vi "Load FLAC.vi"(8 "error in (no error)":errorcluster, 11 "Path":path) -> (0 "error out":errorcluster, 1 "data":waveform(i16)[](array[waveform]), 2 "Sample Rate (Hz)":u32, 3 "Channels":u32, 5 "Length (Samples)":u64)   [LabVIEW 2019, in "LabVIEW Audio Codecs.lvlib"]
doc: "Loads a FLAC file from disk.\n\n<b>Priority:</b> Background priority (lowest)"
uses:
  LabVIEW Audio Codecs.lvlib
  labview_audio_codecs_x86.dll
  labview_audio_codecs_x64.dll
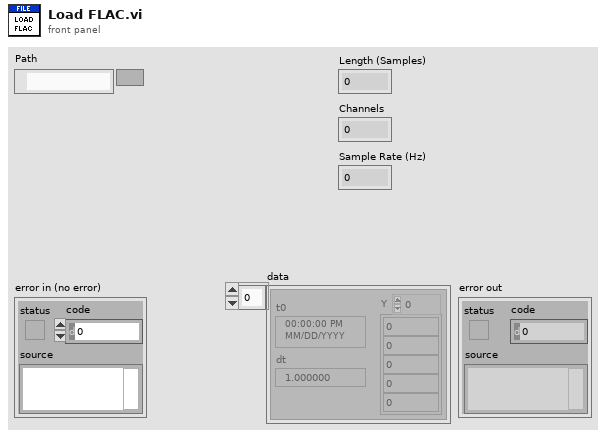
[diagram p1: front panel]
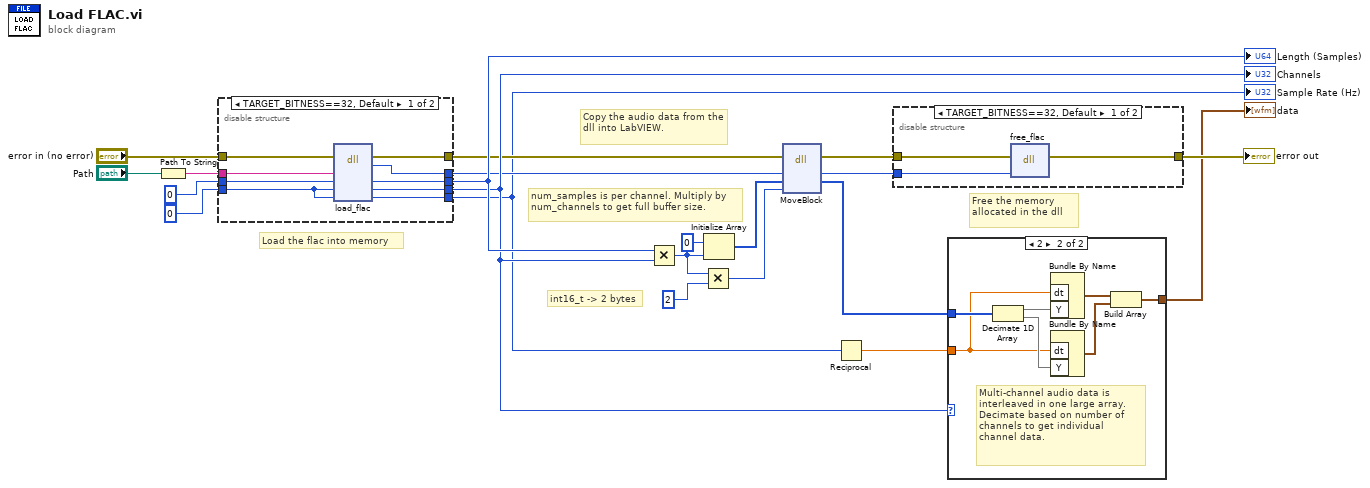
[diagram p0: block diagram]
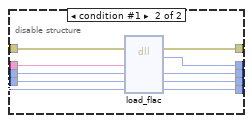
[diagram p2: hidden frame]
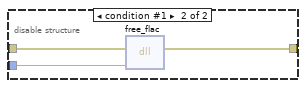
[diagram p3: hidden frame]
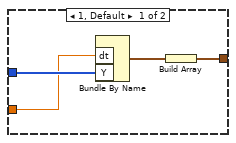
[diagram p4: hidden frame]
diagram:
  # "num_samples is per channel. Multiply by num_channels to get full buffer size."
  # "Free the memory allocated in the dll"
  # "Copy the audio data from the dll into LabVIEW."
  # "Load the flac into memory"
  # "int16_t -> 2 bytes"
  n1 = Path To String(path="Path") -> (string=w15:string)
  n2 = disable-structure shown="TARGET_BITNESS==32, Default" {
    disable-tunnel: "error in (no error)" -> [w30 w39]
    disable-tunnel: [w29 w38] -> w18
    disable-tunnel: [w28 w37] -> w17
    disable-tunnel: [w27 w36] -> w2
    disable-tunnel: w15 -> [w26 w35]
    disable-tunnel: u32 0 ("num_samples") -> [w25 w34]
    disable-tunnel: [w24 w33] -> w12
    disable-tunnel: [w23 w32] -> w10
    disable-tunnel: u64 0 ("num_samples") -> [w22 w31]
    frame condition #0 (active) {
      n3 = dll-call lib="C:/github/dataflowg/labview-simcity-2000-toolkit/src/Sound/LabVIEW Audio Codecs/labview_audio_codecs_x86.*" fn="load_flac"(error in=w30, "file_name"=w26, "num_samples"=w22, "channels"=w25, "sample_rate"=w25) -> (error out=w23:errorcluster, "return type"=w24:i64, "num_samples"=w29:u64, "channels"=w28:u32, "sample_rate"=w27:u32)  [unwired: 3 in, 1 out]
    }
    frame condition #1 {
      n4 = dll-call lib="C:/github/dataflowg/labview-audio-codecs/src/LabVIEW/LabVIEW Audio Codecs/labview_audio_codecs_x64.*" fn="load_flac"(error in=w39, "file_name"=w35, "num_samples"=w31, "channels"=w34, "sample_rate"=w34) -> (error out=w32:errorcluster, "return type"=w33:i64, "num_samples"=w38:u64, "channels"=w37:u32, "sample_rate"=w36:u32)  [unwired: 3 in, 1 out]
    }
  }
  "Length (Samples)" <- w18
  "Channels" <- w17
  "Sample Rate (Hz)" <- w2
  n5 = Multiply(x=w18, y=w17) -> (x*y=w3:u64)
  n6 = Multiply(x=w3, y=u64 2) -> (x*y=w8:u64)
  n7 = Initialize Array(i16 0 ("num_samples"), w3) -> (w11:i16[])
  n8 = dll-call lib="LabVIEW" fn="MoveBlock"(error in=w10, "Address (Pointer)"=w12, "Destination"=w11, "Size"=w8) -> (error out=w6:errorcluster, "Address (Pointer)"=w7:i64, "Destination"=w5:i16[])  [unwired: 4 in, 1 out]
  n9 = Reciprocal(x=w2) -> (1/x=w1:dbl)
  n10 = disable-structure shown="TARGET_BITNESS==32, Default" {
    disable-tunnel: [w42 w45] -> w20
    disable-tunnel: w7 -> [w41 w44]
    disable-tunnel: w6 -> [w40 w43]
    frame condition #0 (active) {
      n11 = dll-call lib="C:/github/dataflowg/labview-simcity-2000-toolkit/src/Sound/LabVIEW Audio Codecs/labview_audio_codecs_x86.*" fn="free_flac"(error in=w40, "Address (Pointer)"=w41) -> (error out=w42:errorcluster)  [unwired: 4 in, 1 out]
    }
    frame condition #1 {
      n12 = dll-call lib="C:/github/dataflowg/labview-audio-codecs/src/LabVIEW/LabVIEW Audio Codecs/labview_audio_codecs_x64.*" fn="free_flac"(error in=w43, "Address (Pointer)"=w44) -> (error out=w45:errorcluster)  [unwired: 4 in, 1 out]
    }
  }
  "error out" <- w20
  n13 = case shown="2" w17 {
    tunnel: w5 -> [w49 w56]
    tunnel: [w48 w51] -> w16
    tunnel: w1 -> [w46 w50]
    frame 1, Default {
      n14 = Bundle By Name("dt"=w46, "Y"=w49) -> (w47:waveform(i16))  [unwired: 1 in]
      n15 = Build Array(w47) -> (w48:waveform(i16)[])
    }
    frame 2 {
      # "Multi-channel audio data is interleaved in one large array. Decimate based on number of channels to get individual channel data."
      n16 = Decimate 1D Array(w56) -> (w55:i16[], w54:i16[])
      n17 = Bundle By Name("dt"=w50, "Y"=w55) -> (w53:waveform(i16))  [unwired: 1 in]
      n18 = Bundle By Name("dt"=w50, "Y"=w54) -> (w52:waveform(i16))  [unwired: 1 in]
      n19 = Build Array(w53, w52) -> (w51:waveform(i16)[])
    }
  }
  "data" <- w16
